vi "AWS-S3-ListObjectsInBucket.vi"(0 "AWS-S3-API in":refnum<class "AWS-S3-API.lvclass">, 5 "Bucket Name":string, 7 "Prefix":string, 11 "error in":errorcluster) -> (4 "AWS-S3-API out":refnum<class "AWS-S3-API.lvclass">, 6 "Objects":T1(array[cluster]), 8 "Subfolders":string[](array[string]), 15 "error out":errorcluster)   [LabVIEW 2012, in "AWS-S3-API.lvclass"]
uses:
  AWS-S3-API.lvclass
  C:/Users/Jack/repo/aws/AWS-SDK/AWSSDK.dll
  repo/aws/AWS-SDK/AWSSDK.dll
panel:
  # "Inputs"
  # "Outputs"
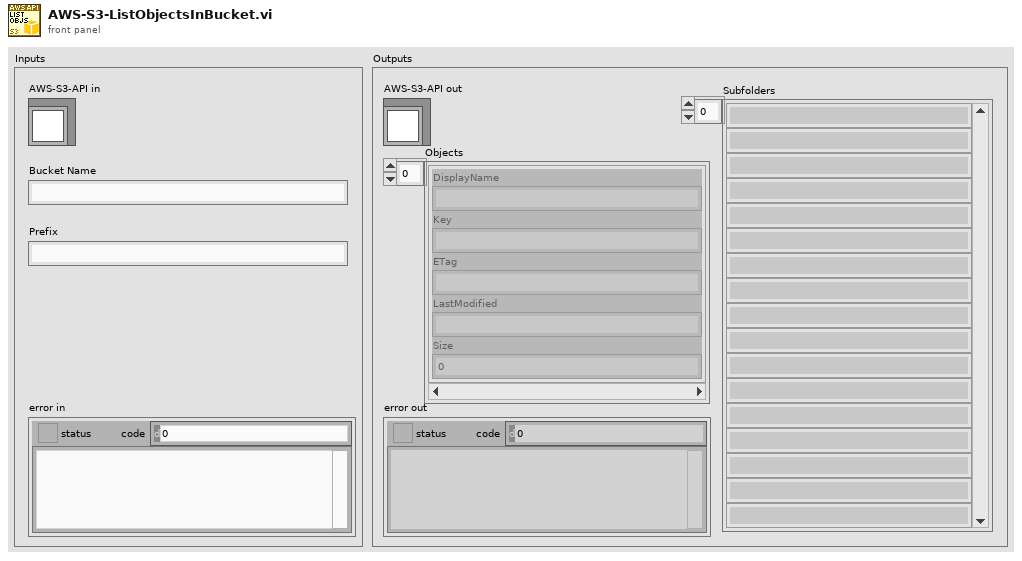
[diagram p1: front panel]
types:
  T1 = cluster{"DisplayName":string, "Key":string, "ETag":string, "LastModified":string, "Size":i64}[]
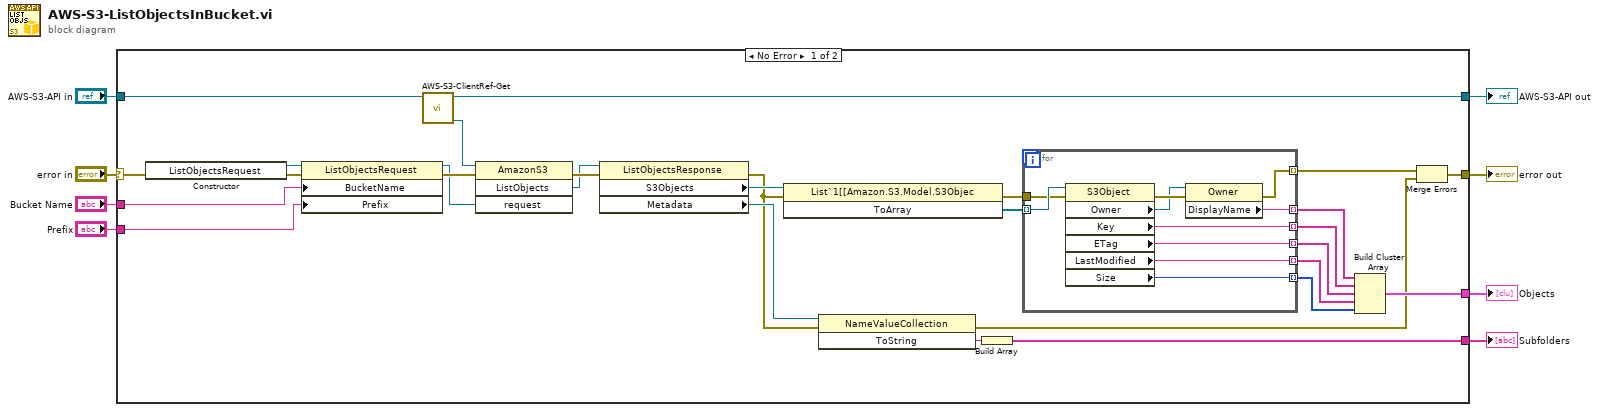
[diagram p0: block diagram]
diagram:
  n1 = case shown="No Error" "error in" {
    selector: "error in" -> [w33 w48]
    tunnel: [w28 w48] -> w8
    tunnel: [w9 w47] -> w6
    tunnel: "AWS-S3-API in" -> [w10 w47]
    tunnel: "Bucket Name" -> [w14 _]
    tunnel: [w22 _] -> w3
    tunnel: [w19 _] -> w2
    tunnel: "Prefix" -> [w13 _]
    frame No Error {
      n2 = constructor class="ListObjectsRequest"(error in=w33) -> (reference out=w18:refnum<k24>, error out=w17:errorcluster)  [unwired: 2 in, 1 out]
      n3 = property class="ListObjectsRequest"(reference=w18, error in=w17, "BucketName"=w14, "Prefix"=w13) -> (reference out=w15:refnum<k24>, error out=w16:errorcluster)
      n4 = call "AWS-S3-ClientRef-Get.vi"("AWS-S3-API"=w10) -> ("S3 Client ref"=w11:refnum<k24>, "AWS-S3-API out"=w9:refnum<class "AWS-S3-API.lvclass">)  [unwired: 9 in]
      n5 = invoke class="AmazonS3" method="ListObjects"(reference=w11, error in=w16, "request"=w15) -> (error out=w32:errorcluster, "ListObjects"=w12:refnum<k24>)  [unwired: 1 in, 2 out]
      n6 = property class="ListObjectsResponse"(reference=w12, error in=w32) -> (error out=w31:errorcluster, "S3Objects"=w36:refnum<k24>, "Metadata"=w34:refnum<k24>)  [unwired: 1 out]
      n7 = invoke class="List`1[[Amazon.S3.Model.S3Objec" method="ToArray"(reference=w36, error in=w31) -> (error out=w30:errorcluster, "ToArray"=w35:refnum<k24>[])  [unwired: 1 in, 1 out]
      n8 = invoke class="NameValueCollection" method="ToString"(reference=w34, error in=w31) -> (error out=w20:errorcluster, "ToString"=w21:string)  [unwired: 1 in, 1 out]
      n9 = Build Array(w21) -> (w19:string[])
      n10 = for {
        tunnel: w35 -> [w46] mode=indexing
        tunnel: w30 -> [w45]
        tunnel: [w42] -> w27 mode=indexing
        tunnel: [w41] -> w29 mode=indexing
        tunnel: [w40] -> w26 mode=indexing
        tunnel: [w39] -> w25 mode=indexing
        tunnel: [w38] -> w24 mode=indexing
        tunnel: [w37] -> w23 mode=indexing
        n11 = property class="S3Object"(reference=w46, error in=w45) -> (error out=w44:errorcluster, "Owner"=w43:refnum<k24>, "Key"=w40:string, "ETag"=w39:string, "LastModified"=w38:string, "Size"=w37:i64)  [unwired: 1 out]
        n12 = property class="Owner"(reference=w43, error in=w44) -> (error out=w41:errorcluster, "DisplayName"=w42:string)  [unwired: 1 out]
      }
      n13 = Build Cluster Array(w27, w26, w25, w24, w23) -> (w22:T1)
      n14 = Merge Errors(w29, w20) -> (w28:errorcluster)
    }
    frame Error {
    }
  }
  "error out" <- w8
  "AWS-S3-API out" <- w6
  "Objects" <- w3
  "Subfolders" <- w2
